vi "Convert Image Options to U32.vi"(1 "Options":T1 {"GI_HEADMASK" max=15}) -> (0 "result":u32)   [LabVIEW 2013, in "VRI.lvlib"]
doc: "This VI is used to process the image options such that it is formated as a U32."
uses:
  VRI.lvlib
  _Type Defs/GetImage Options.ctl
panel:
  out "Boolean array":bool[](array[boolean])
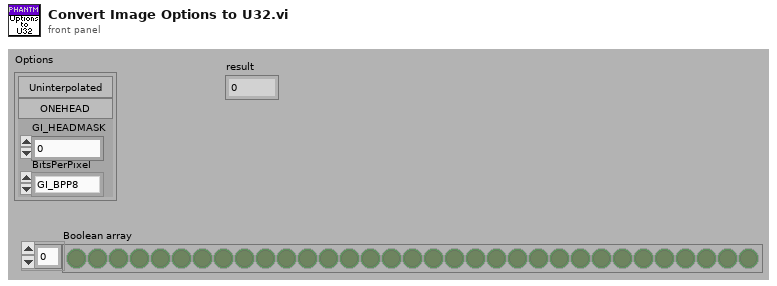
[diagram p1: front panel]
types:
  T1 = typedef "VRI.lvlib/GetImage Options.ctl" = cluster{"GI_INTERPOLATED":bool, "GI_ONEHEAD":bool, "GI_HEADMASK":u8, "BitsPerPixel":enum32{"GI_BPP8", "GI_PACKED", "GI_BPP16"}}
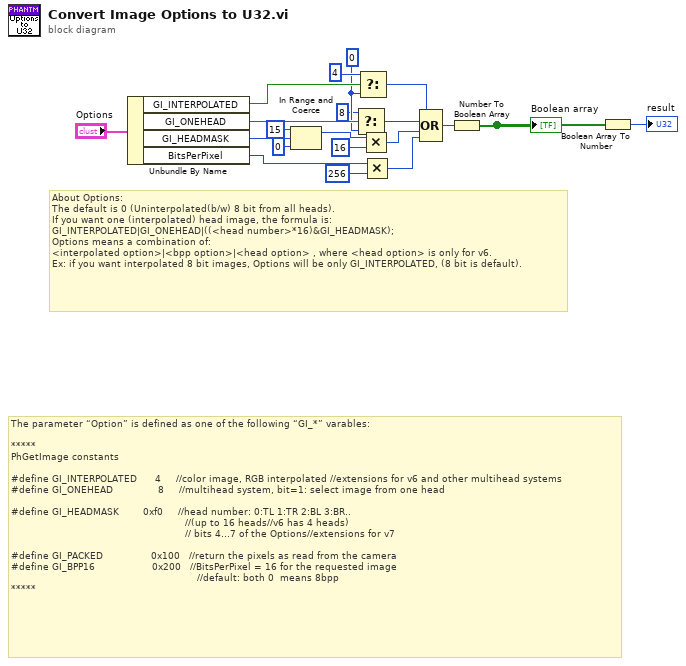
[diagram p0: block diagram]
diagram:
  w16 = u32 0 ("f")
  # "The parameter “Option” is defined as one of the following “GI_*” varables:\n\n*****\nPhGetImage constants\n\n#define GI_INTERPOLATED      4     //color image, RGB interpolated //extensions for v6 and other multihead systems\n#define GI_ONEHEAD               8     //multihead system, bit=1: select image from one head \n\n#define GI_HEADMASK        0xf0     //head number: 0:TL 1:TR 2:BL 3:BR..\n                                                          //(up to 16 heads//v6 has 4 heads)\n                                                          // bits 4...7 of the Options//extensions for v7 \n\n#define GI_PACKED                0x100   //return the pixels as read from the camera \n#define GI_BPP16                   0x200   //BitsPerPixel = 16 for the requested image \n                                                              //default: both 0  means 8bpp\n*****"
  # "About Options:\nThe default is 0 (Uninterpolated(b/w) 8 bit from all heads). \nIf you want one (interpolated) head image, the formula is:\nGI_INTERPOLATED|GI_ONEHEAD|((<head number>*16)&GI_HEADMASK);\nOptions means a combination of:\n<interpolated option>|<bpp option>|<head option> , where <head option> is only for v6.\nEx: if you want interpolated 8 bit images, Options will be only GI_INTERPOLATED, (8 bit is default)."
  n1 = Unbundle By Name("Options") -> ("GI_INTERPOLATED"=w18:bool, "GI_ONEHEAD"=w17:bool, "GI_HEADMASK"=w10:u8, "BitsPerPixel"=w9:enum32{"GI_BPP8", "GI_PACKED", "GI_BPP16"})
  n2 = In Range and Coerce(upper limit=u8 15, x=w10, lower limit=u8 0) -> (coerced(x)=w6:u8)  [unwired: 1 out]
  n3 = Select(t=u32 8, s=w17, f=w16) -> (s? t:f=w11:u32)
  n4 = Select(t=u32 4, s=w18, f=w16) -> (s? t:f=w12:u32)
  n5 = Multiply(x=w6, y=u32 16) -> (x*y=w8:u32)
  n6 = Multiply(x=w9, y=u32 256) -> (x*y=w7:u32)
  n7 = Compound Arithmetic op=OR(w12, w11, w8, w7) -> (w3:u32)
  n8 = Number To Boolean Array(number=w3) -> (Boolean array=w1:bool[])
  "Boolean array" <- w1
  n9 = Boolean Array To Number(Boolean array=w1) -> (number=→"result":u32)
